vi "JSAxiesToString.vi"(0 "JS ID":i32, 1 "Cluster":cluster{"X Axis":dbl, "Y Axis":dbl}, 3 "error in (no error)":errorcluster) -> (7 "Axies Out":string, 10 "error out":errorcluster)   [LabVIEW 2012]
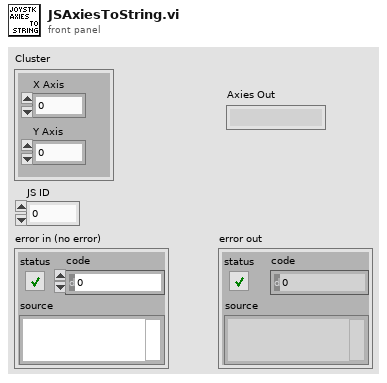
[diagram p1: front panel]
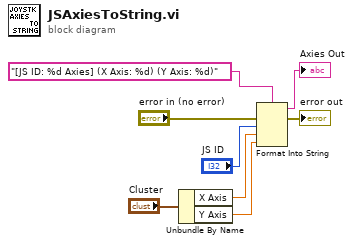
[diagram p0: block diagram]
diagram:
  n1 = Unbundle By Name("Cluster") -> ("X Axis"=w7:dbl, "Y Axis"=w6:dbl)
  n2 = Format Into String(format string="[JS ID: %d Axies] (X Axis: %d) (Y Axis: %d)", error in="error in (no error)", "JS ID", w7, w6) -> (resulting string=→"Axies Out":string, error out=→"error out":errorcluster)  [unwired: 1 in]
